vi "Initialize.vi"(8 "error in":errorcluster, 10 "parameters":variant, 11 "group in":refnum<class "cfg group.lvclass">) -> (0 "error out":errorcluster, 2 "summary":T2[](array[typedef]), 3 "data value reference":T1)   [LabVIEW 2013, in "cfg group.lvclass"]
doc: "This Vi initializes the data of a node its default state.\nThe object is not created inside of this ViI, beacuase it is created from a File depending on user selection."
uses:
  cfg group.lvclass
  CEF_TreeControl/Node/Summary.ctl
  CEF_TreeControl/Node/NodeRef.ctl
  CEF_TreeControl/Node/NISE_CEF_Node.lvclass
  groupcfg/group configuration.lvclass
  cfg group.lvclass/cfg group.ctl
  CEF_TreeControl/serializable node/NISE_CEF_serializable node.lvclass
  groupcfg/Write groupName.vi
  CEF_TreeControl/serializable configuration/set metadata property.vi
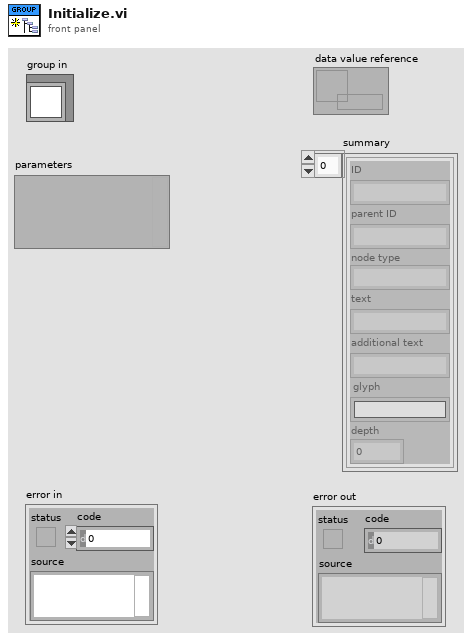
[diagram p1: front panel]
types:
  T1 = typedef "NISE_CEF_Node.lvclass/NodeRef.ctl" = refnum<data-value>
  T2 = typedef "NISE_CEF_Node.lvclass/Summary.ctl" = cluster{"ID":string, "parent ID":string, "node type":string, "text":string, "additional text":string, "glyph":string, "depth":i32}
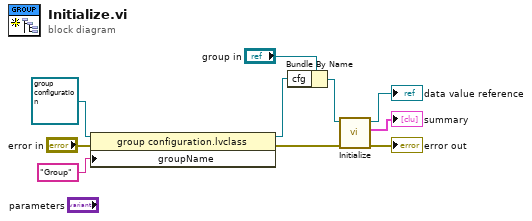
[diagram p0: block diagram]
diagram:
  n1 = property class="group configuration.lvclass"(reference=refnum<class "group configuration.lvclass"> refnum ("group configuration.lvclass"), error in="error in", "groupName"="Group") -> (reference out=w2:refnum<class "group configuration.lvclass">, error out=w4:errorcluster)
  n2 = Bundle By Name(cluster="group in", "cfg"=w2) -> (w5:refnum<class "cfg group.lvclass">)
  n3 = call-parent "Initialize.vi"("error in"=w4, "node in"=w5) -> ("error out"=→"error out":errorcluster, "summary"=→"summary":T2[], "data value reference"=→"data value reference":T1)  [unwired: 7 in]
